vi "Read Descriptor.vi"(8 "error in (no error)":errorcluster, 11 "LakeShore 340 in":refnum<class "LakeShore 340.lvclass">) -> (0 "error out":errorcluster, 2 "Class Descriptor":string="LakeShore 340", 3 "LakeShore 340 out":refnum<class "LakeShore 340.lvclass">)   [LabVIEW 2015, in "LakeShore 340.lvclass"]
uses:
  LakeShore 340.lvclass
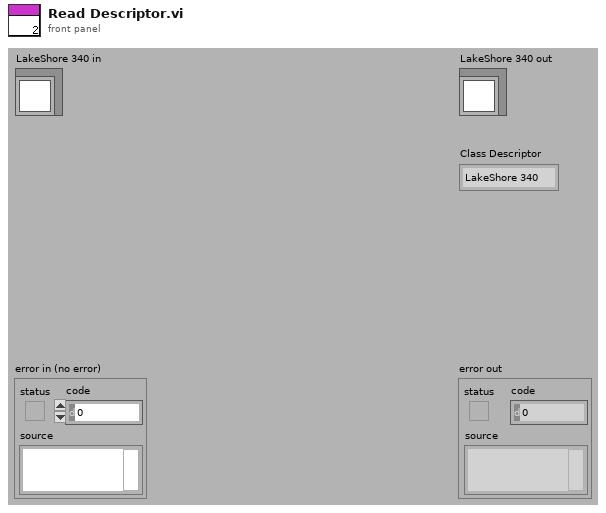
[diagram p1: front panel]
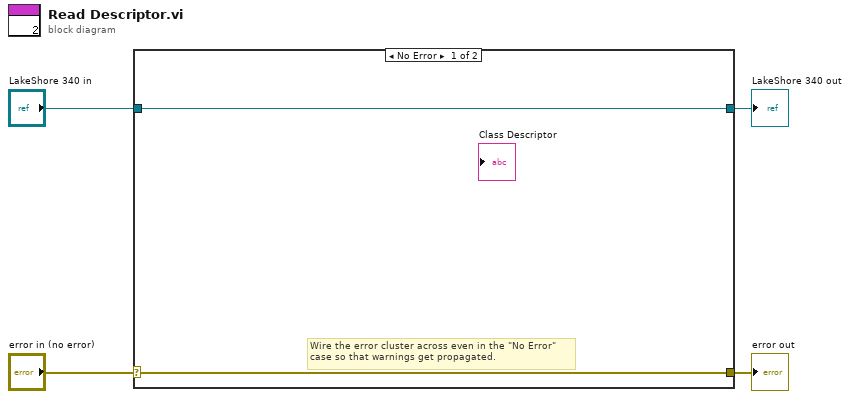
[diagram p0: block diagram]
diagram:
  n1 = case shown="No Error" "error in (no error)" {
    selector: "error in (no error)" -> [w5 w8]
    tunnel: [w5 w8] -> w3
    tunnel: [w6 w7] -> w1
    tunnel: "LakeShore 340 in" -> [w6 w7]
    frame No Error {
      # "Wire the error cluster across even in the \"No Error\"\ncase so that warnings get propagated."
    }
    frame Error {
    }
  }
  "error out" <- w3
  "LakeShore 340 out" <- w1
